vi "GlobalAlloc.vi"(4 "error in (no error)":errorcluster, 6 "uFlags":T1(ring), 7 "Bytes (0)":i32) -> (0 "error out":errorcluster, 3 "hMem":i32 format="%.0x")   [LabVIEW 2011]
uses:
  KERNEL32.DLL
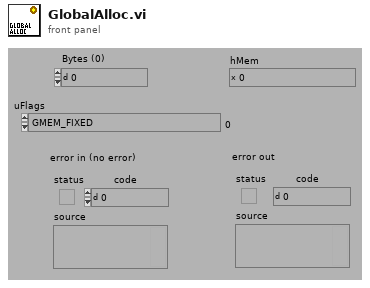
[diagram p1: front panel]
types:
  T1 = enum16{"GMEM_FIXED", "GMEM_MOVEABLE", "GMEM_NOCOMPACT", "GMEM_NODISCARD", "GMEM_ZEROINIT", "GMEM_MODIFY", "GMEM_DISCARDABLE", "GMEM_NOT_BANKED", "GMEM_SHARE", "GMEM_DDESHARE", "GMEM_NOTIFY", "GMEM_LOWER", "GMEM_VALID_FLAGS", "GMEM_INVALID_HANDLE", "GHND", "GPTR"}
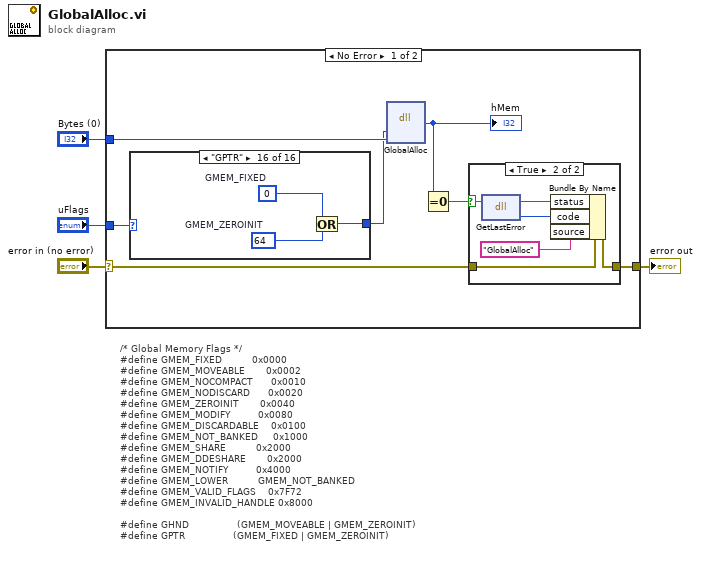
[diagram p0: block diagram]
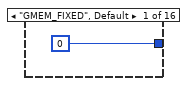
[diagram p2: hidden frame]
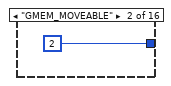
[diagram p3: hidden frame]
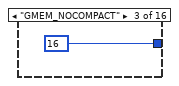
[diagram p4: hidden frame]
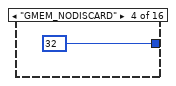
[diagram p5: hidden frame]
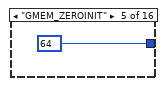
[diagram p6: hidden frame]
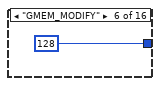
[diagram p7: hidden frame]
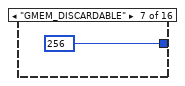
[diagram p8: hidden frame]
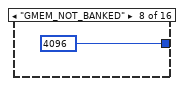
[diagram p9: hidden frame]
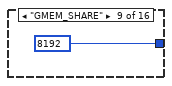
[diagram p10: hidden frame]
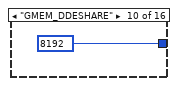
[diagram p11: hidden frame]
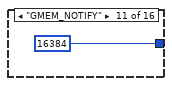
[diagram p12: hidden frame]
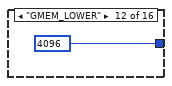
[diagram p13: hidden frame]
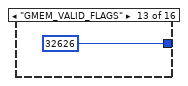
[diagram p14: hidden frame]
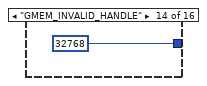
[diagram p15: hidden frame]
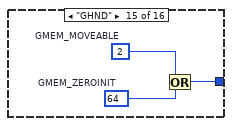
[diagram p16: hidden frame]
diagram:
  # "/* Global Memory Flags */\n#define GMEM_FIXED          0x0000\n#define GMEM_MOVEABLE       0x0002\n#define GMEM_NOCOMPACT      0x0010\n#define GMEM_NODISCARD      0x0020\n#define GMEM_ZEROINIT       0x0040\n#define GMEM_MODIFY         0x0080\n#define GMEM_DISCARDABLE    0x0100\n#define GMEM_NOT_BANKED     0x1000\n#define GMEM_SHARE          0x2000\n#define GMEM_DDESHARE       0x2000\n#define GMEM_NOTIFY         0x4000\n#define GMEM_LOWER          GMEM_NOT_BANKED\n#define GMEM_VALID_FLAGS    0x7F72\n#define GMEM_INVALID_HANDLE 0x8000\n\n#define GHND                (GMEM_MOVEABLE | GMEM_ZEROINIT)\n#define GPTR                (GMEM_FIXED | GMEM_ZEROINIT)"
  n1 = case shown="No Error" "error in (no error)" {
    selector: "error in (no error)" -> [w9 w38]
    tunnel: [w8 w38] -> w3
    tunnel: "Bytes (0)" -> [w7 _]
    tunnel: "uFlags" -> [w6 _]
    frame No Error {
      n2 = case shown="\"GPTR\"" w6 {
        tunnel: [u32 0 ("uFlags") u32 2 ("uFlags") u32 16 ("uFlags") u32 32 ("uFlags") u32 64 ("uFlags") u32 128 ("uFlags") u32 256 ("uFlags") u32 4096 ("uFlags") u32 8192 ("uFlags") u32 8192 ("uFlags") u32 16384 ("uFlags") u32 4096 ("uFlags") u32 32626 ("uFlags") u32 32768 ("uFlags") w28 w31] -> w5
        frame "GMEM_FIXED", Default {
        }
        frame "GMEM_MOVEABLE" {
        }
        frame "GMEM_NOCOMPACT" {
        }
        frame "GMEM_NODISCARD" {
        }
        frame "GMEM_ZEROINIT" {
        }
        frame "GMEM_MODIFY" {
        }
        frame "GMEM_DISCARDABLE" {
        }
        frame "GMEM_NOT_BANKED" {
        }
        frame "GMEM_SHARE" {
        }
        frame "GMEM_DDESHARE" {
        }
        frame "GMEM_NOTIFY" {
        }
        frame "GMEM_LOWER" {
        }
        frame "GMEM_VALID_FLAGS" {
        }
        frame "GMEM_INVALID_HANDLE" {
        }
        frame "GHND" {
          w26 = u32 64  # GMEM_ZEROINIT
          w27 = u32 2  # GMEM_MOVEABLE
          n3 = Or(x=w27, y=w26) -> (x .or. y?=w28:u32)
        }
        frame "GPTR" {
          w29 = u32 64  # GMEM_ZEROINIT
          w30 = u32 0  # GMEM_FIXED
          n4 = Or(x=w30, y=w29) -> (x .or. y?=w31:u32)
        }
      }
      n5 = dll-call lib="KERNEL32.DLL" fn="GlobalAlloc" label="long GlobalAlloc(\n     unsigned long uFlags, unsigned long dwBytes);"("uFlags"=w5, "dwBytes"=w7) -> ("hMem"=w11:i32)  [unwired: 5 in, 2 out]
      "hMem" <- w11
      n6 = Equal To 0?(x=w11) -> (x = 0?=w10:bool)
      n7 = case shown="True" w10 {
        selector: w10 -> [_ w36]
        tunnel: w9 -> [w32 w37]
        tunnel: [w32 w35] -> w8
        frame False {
        }
        frame True {
          n8 = dll-call lib="KERNEL32.DLL" fn="GetLastError"() -> (w34:i32)  [unwired: 3 in, 2 out]
          n9 = Bundle By Name(cluster=w37, "status"=w36, "code"=w34, "source"="GlobalAlloc") -> (w35:errorcluster)
        }
      }
    }
    frame Error {
    }
  }
  "error out" <- w3
